vi "Pixel 1 Condition (SubVI).vi"(10 "Contour Scan in":T1) -> (2 "Contour Scan out":T1)   [LabVIEW 2015]
uses:
  Controls (FPGA)/Contour Scan.ctl
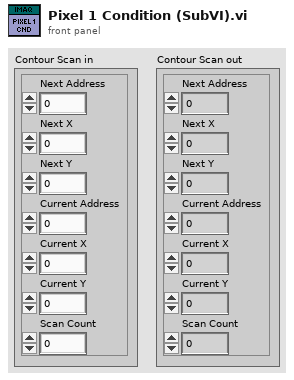
[diagram p1: front panel]
types:
  T1 = typedef "Contour Scan.ctl" = cluster{"Next Address":fxp<+,24,24>, "Next X":fxp<+,12,12>, "Next Y":fxp<+,12,12>, "Current Address":fxp<+,24,24>, "Current X":fxp<+,12,12>, "Current Y":fxp<+,12,12>, "Scan Count":u32}
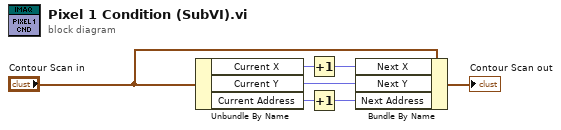
[diagram p0: block diagram]
diagram:
  n1 = Unbundle By Name("Contour Scan in") -> ("Current X"=w5:fxp<+,12,12>, "Current Y"=w4:fxp<+,12,12>, "Current Address"=w2:fxp<+,24,24>)
  n2 = Increment(x=w5) -> (x+1=w6:fxp<+,12,12>)
  n3 = Increment(x=w2) -> (x+1=w3:fxp<+,24,24>)
  n4 = Bundle By Name(cluster="Contour Scan in", "Next X"=w6, "Next Y"=w4, "Next Address"=w3) -> (→"Contour Scan out":T1)
